vi "Ev Cmd Save Data File.vi"(8 "error in (no error)":errorcluster, 11 "LF2R IDE in":refnum<class "LF2R IDE.lvclass">) -> (0 "error out":errorcluster, 3 "LF2R IDE out":refnum<class "LF2R IDE.lvclass">)   [LabVIEW 2018, in "LF2R IDE.lvlib" / "LF2R IDE.lvclass"]
uses:
  LF2R IDE.lvclass
  LF2R IDE.lvclass/LF2R IDE.ctl
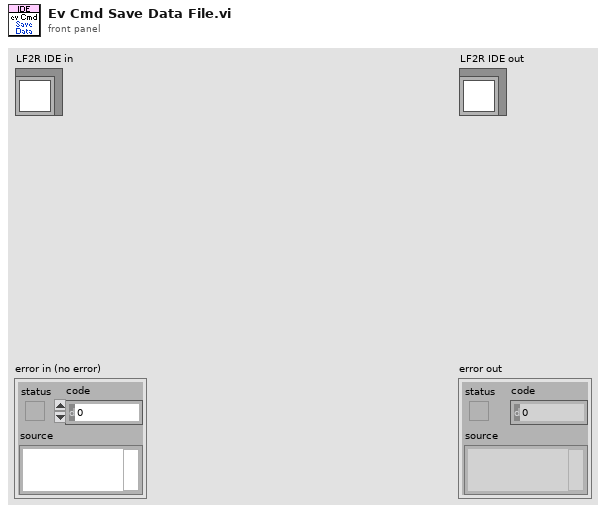
[diagram p1: front panel]
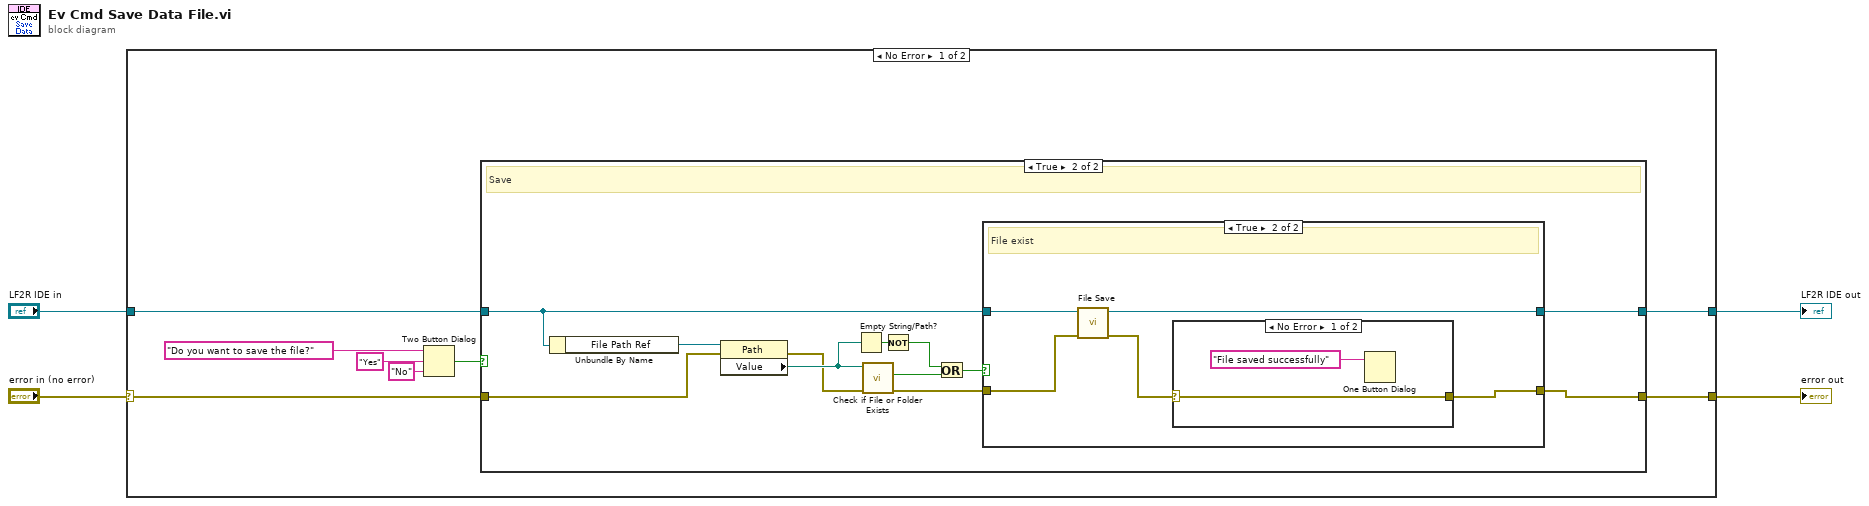
[diagram p0: block diagram]
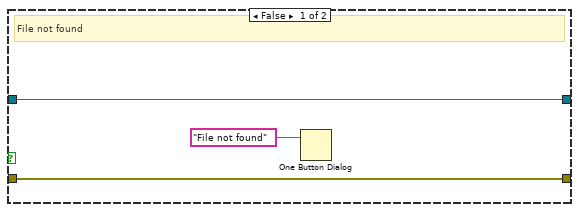
[diagram p3: hidden frame]
diagram:
  n1 = case shown="No Error" "error in (no error)" {
    selector: "error in (no error)" -> [w5 w39]
    tunnel: [w12 w39] -> w1
    tunnel: [w10 w38] -> w2
    tunnel: "LF2R IDE in" -> [w11 w38]
    frame No Error {
      n2 = Two Button Dialog(message="Do you want to save the file?", 1:"No" ("F button name (\"Cancel\")"), 2:"Yes" ("T button name (\"OK\")")) -> (T button?=w6:bool)
      n3 = case shown="True" w6 {
        tunnel: [w13 w26] -> w12
        tunnel: w11 -> [w14 w18]
        tunnel: [w14 w25] -> w10
        tunnel: w5 -> [w13 w17]
        frame False {
        }
        frame True {
          # "Save"
          n4 = Unbundle By Name(w18) -> ("File Path Ref"=w24:refnum<vi>)
          n5 = property class="Path"(reference=w24, error in=w17) -> (error out=w21:errorcluster, "Value"=w22:path)  [unwired: 1 out]
          n6 = Empty String/Path?(string/path=w22) -> (empty?=w23:bool)
          n7 = call <vilib>:"Check if File or Folder Exists.vi"("error in (no error)"=w21, "path"=w22) -> ("error out"=w16:errorcluster, "file or folder exists?"=w20:bool)  [unwired: 7 in, 1 out]
          n8 = Not(x=w23) -> (.not. x?=w19:bool)
          n9 = Or(x=w19, y=w20) -> (x .or. y?=w15:bool)
          n10 = case shown="True" w15 {
            tunnel: [w27 w34] -> w26
            tunnel: [w28 w33] -> w25
            tunnel: w18 -> [w28 w31]
            tunnel: w16 -> [w27 w30]
            frame False {
              # "File not found"
              n11 = One Button Dialog(message="File not found") -> ()  [unwired: 1 in, 1 out]
            }
            frame True {
              # "File exist"
              n12 = call "File Save.vi"("error in (no error)"=w30, "LF2R IDE in"=w31) -> ("error out"=w32:errorcluster, "LF2R IDE out"=w33:refnum<class "LF2R IDE.lvclass">)  [unwired: 7 in, 1 out]
              n13 = case shown="No Error" w32 {
                selector: w32 -> [w35 w37]
                tunnel: [w35 w37] -> w34
                frame No Error {
                  n14 = One Button Dialog(message="File saved successfully") -> ()  [unwired: 1 in, 1 out]
                }
                frame Error {
                }
              }
            }
          }
        }
      }
    }
    frame Error {
    }
  }
  "error out" <- w1
  "LF2R IDE out" <- w2
